vi "Clear Temporary Variables.vi"(6 "Backend engine":T1, 8 "error in":errorcluster) -> (0 "error out":errorcluster)   [LabVIEW 2013, in "QWTBLVLib.lvlib"]
doc: "Clears variables in Matlab created by this library."
uses:
  QWTBLVLib.lvlib
  TD Backend Engine.ctl
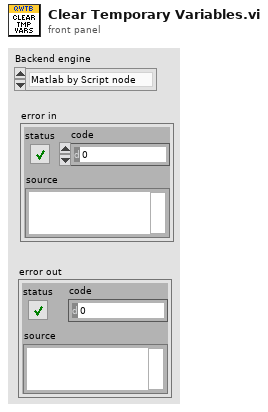
[diagram p1: front panel]
types:
  T1 = typedef "QWTBLVLib.lvlib/TD Backend Engine.ctl" = enum16{"Matlab by Script node", "GNU Octave by GOLPI"}
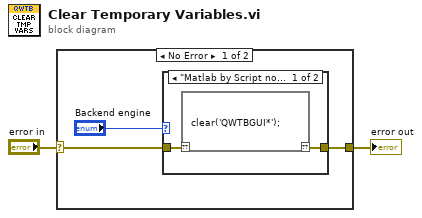
[diagram p0: block diagram]
diagram:
  n1 = case shown="No Error" "error in" {
    selector: "error in" -> [w4 w9]
    tunnel: [w5 w9] -> w2
    frame No Error {
      n2 = case shown="\"Matlab by Script node\", Default" "Backend engine" {
        tunnel: [w7 w8] -> w5
        tunnel: w4 -> [w6 w8]
        frame "Matlab by Script node", Default {
          n3 = script code="clear('QWTBGUI*');"("??"=w6) -> ("??"=w7:errorcluster)
        }
        frame "GNU Octave by GOLPI" {
          # "#2do"
        }
      }
    }
    frame Error {
    }
  }
  "error out" <- w2
